vi "Modify Numeric Rep in VI (Array).vi"(8 "error in":errorcluster, 10 "Numeric Representation Param":T1[](array[typedef]), 11 "Original VI":path=path "C:/Users/OneEd/OneDrive/Desktop/MicroPort Job/CTDB/src/db_script/DB Select Template.vi") -> (0 "error out":errorcluster, 3 "Save as out":path=path "C:/Users/OneEd/OneDrive/Desktop/MicroPort Job/CTDB/src/db_script/DB Select Template.vi")   [LabVIEW 2021, in "EDT VI Script.lvlib"]
uses:
  EDT VI Script.lvlib
  Modify Numeric Representation Param.ctl
  <vilib>/numeric/LVNumericRepresentation.ctl
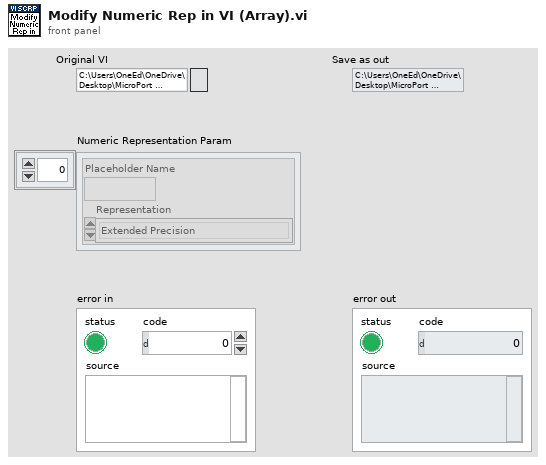
[diagram p1: front panel]
types:
  T1 = typedef "EDT VI Script.lvlib/Modify Numeric Representation Param.ctl" = cluster{"Placeholder Name":string, "Numeric Representation":T2}
  T2 = typedef "LVNumericRepresentation.ctl" = enum32{"Extended Precision", "Double Precision", "Single Precision", "Long", "Word", "Byte", "Unsigned Long", "Unsigned Word", "Unsigned Byte", "Complex Extended", "Complex Double", "Complex Single", "Quad", "Unsigned Quad", "Fixed-Point"}
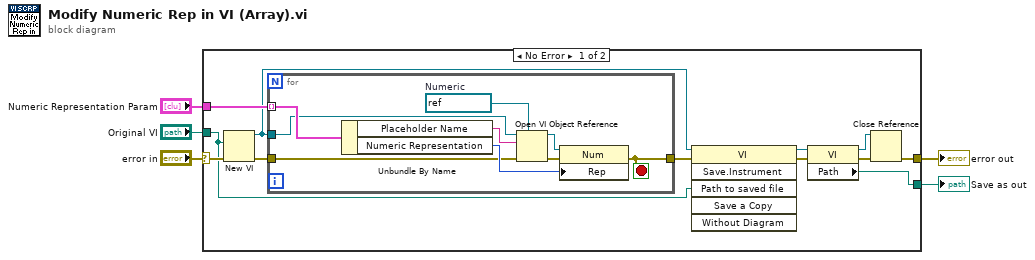
[diagram p0: block diagram]
diagram:
  n1 = case shown="No Error" "error in" {
    selector: "error in" -> [w16 w28]
    tunnel: [w6 w28] -> w4
    tunnel: "Numeric Representation Param" -> [w17 _]
    tunnel: "Original VI" -> [w9 w27]
    tunnel: [w7 w27] -> w1
    frame No Error {
      n2 = New VI(8:w16, 10:w9) -> (0:w15:errorcluster, 3:w8:refnum<vi>)  [unwired: 5 in]
      n3 = for {
        tunnel: w17 -> [w26] mode=indexing
        tunnel: w8 -> [w19]
        tunnel: w15 -> [w20]
        tunnel: [w18] -> w10
        stop <- w18 stop-if-true
        w23 = refnum<vi> refnum  # Numeric
        n4 = Unbundle By Name(w26) -> ("Placeholder Name"=w25:string, "Numeric Representation"=w22:T2)
        n5 = Open VI Object Reference(7:w23, 8:w20, 10:w25, 11:w19) -> (0:w24:errorcluster, 3:w21:refnum<vi>)
        n6 = property class="Num"(reference=w21, error in=w24, "Rep"=w22) -> (error out=w18:errorcluster)  [unwired: 1 out]
      }
      n7 = invoke class="VI" method="Save.Instrument"(reference=w8, error in=w10, "Path to saved file"=w9) -> (reference out=w12:refnum<vi>, error out=w11:errorcluster)  [unwired: 3 in, 4 out]
      n8 = property class="VI"(reference=w12, error in=w11) -> (reference out=w14:refnum<vi>, error out=w13:errorcluster, "Path"=w7:path)
      n9 = Close Reference(reference=w14, error in (no error)=w13) -> (error out=w6:errorcluster)
    }
    frame Error {
    }
  }
  "error out" <- w4
  "Save as out" <- w1
